vi "Graph.vi"() -> ()   [LabVIEW 2016, in "PanelDataNode.lvclass"]
uses:
  PanelDataNode.lvclass
  PanelObject/PanelObject.lvclass
  PanelDataNode.lvclass/PanelDataNode.ctl
  Split Mode.ctl
  <vilib>/Analysis/baseanly.llb/Mean (DBL).vi
  <vilib>/measure/NI_MABase.lvlib
  <vilib>/Analysis/NI_AALBase.lvlib
panel:
  out "波形图表":waveform(dbl)(graph)={"t0"=timestamp(9406.0 s since 1904-01-01), "dt"=0.001, "Y"=array[1000 elements]}
  in  "Node*":refnum<data-value>
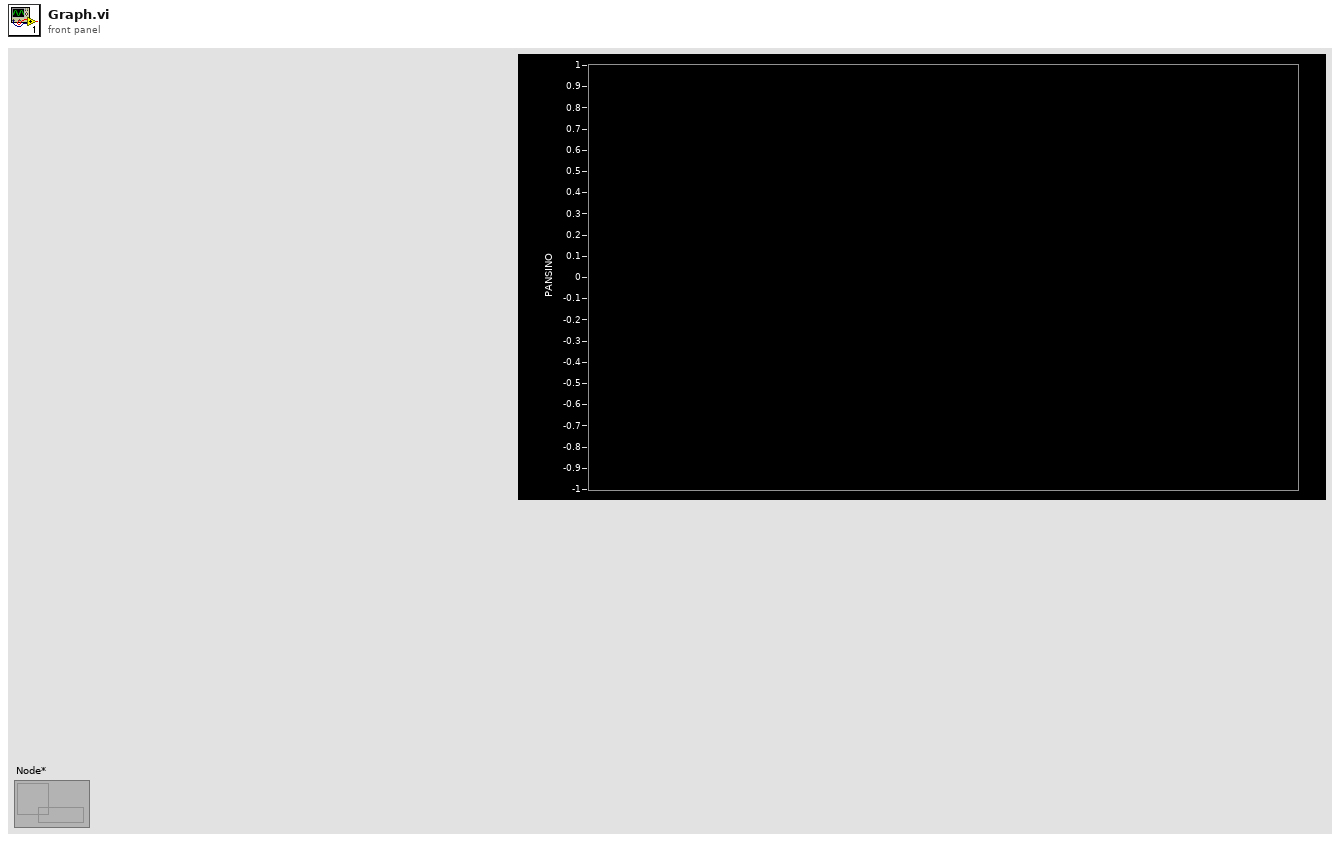
[diagram p1: front panel]
types:
  T1 = enum16{"Sine Wave", "Triangle Wave", "Square Wave", "Sawtooth Wave"}
  T2 = typedef "PanelDataNode.lvclass/Split Mode.ctl" = enum16{"Horizontal(up)", "Vertical(left)", "Horizontal(down)", "Vertical(right)"}
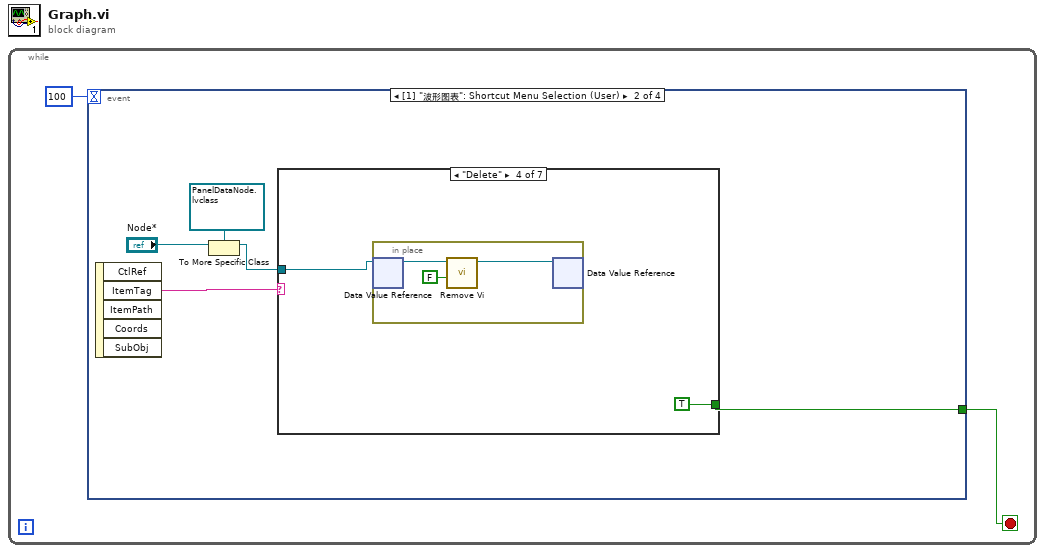
[diagram p0: block diagram]
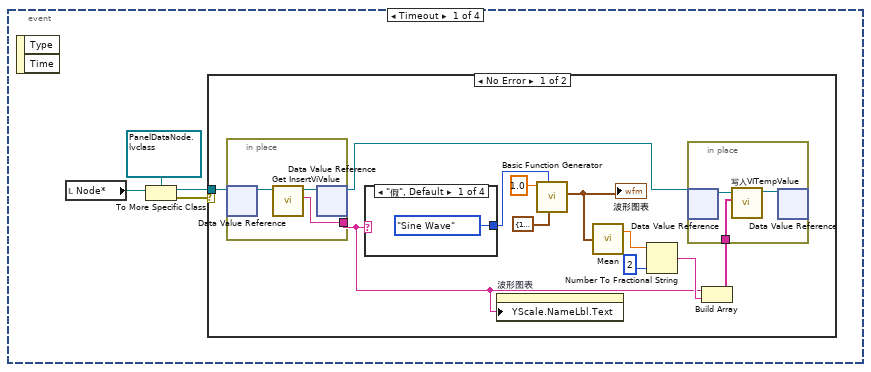
[diagram p2: hidden frame]
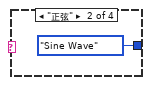
[diagram p3: hidden frame]
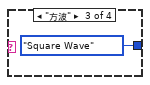
[diagram p4: hidden frame]
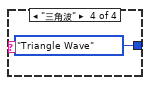
[diagram p5: hidden frame]
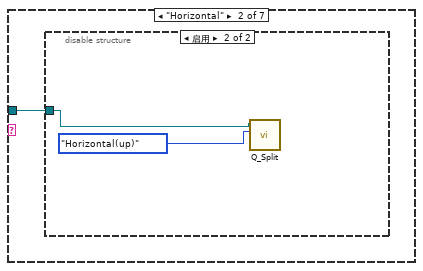
[diagram p8: hidden frame]
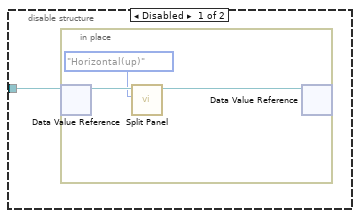
[diagram p9: hidden frame]
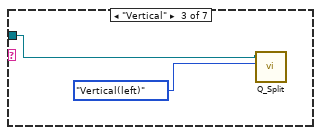
[diagram p10: hidden frame]
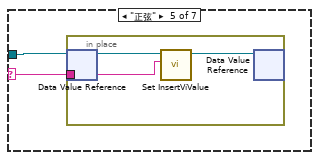
[diagram p11: hidden frame]
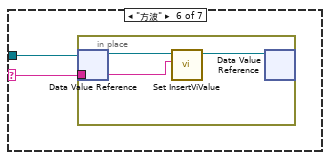
[diagram p12: hidden frame]
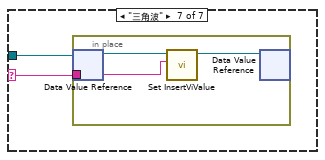
[diagram p13: hidden frame]
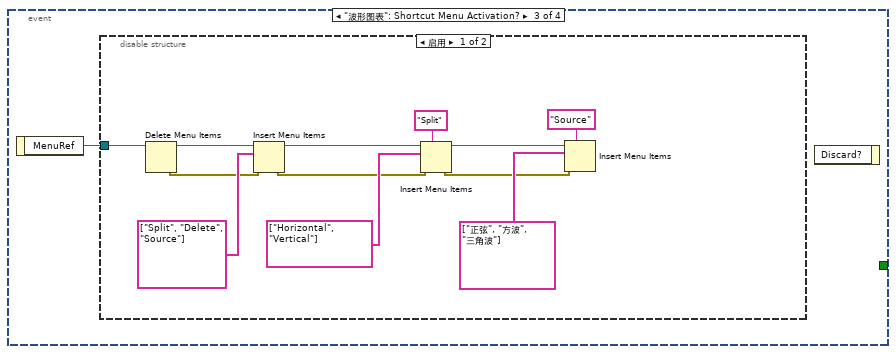
[diagram p14: hidden frame]
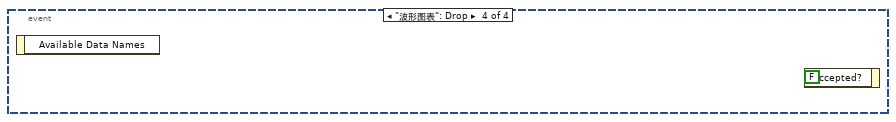
[diagram p16: hidden frame]
diagram:
  n1 = while {
    stop <- w1 stop-if-true
    n2 = event shown="[1] \"波形图表\": Shortcut Menu Selection (User)" {
      selector: _ -> [_ _ _ _]
      dyn-events: _ -> [_ _ _ _]
      timeout: 100 -> [_ _ _ _]
      tunnel: [_ w28 _ _] -> w1
      event Timeout {
        n3 = event-data() -> ()  [unwired: 1 in, 2 out]
        n4 = local read "Node*"() -> (w5:refnum<data-value>)
        n5 = To More Specific Class(target class=refnum<data-value> refnum ("Node*"), reference=w5) -> (specific class reference=w3:refnum<data-value>, error out=w4:errorcluster)  [unwired: 1 in]
        n6 = case shown="No Error" w4 {
          tunnel: w3 -> [w15 _]
          frame No Error {
            n7 = in-place {
              in-place-border: [w25] -> w7
              n8 = in-place-dvr #1(w15) -> (w27:refnum<class "PanelDataNode.lvclass">)  [unwired: 1 out]
              n9 = call-dynamic "Get InsertViValue.vi"("PanelDataNode 输入"=w27) -> ("ViValue"=w25:string, "PanelDataNode 输出"=w26:refnum<class "PanelDataNode.lvclass">)  [unwired: 8 in, 1 out]
              n10 = in-place-dvr #1(w26) -> (w12:refnum<data-value>)  [unwired: 1 out]
            }
            n11 = case shown="\"假\", Default" w7 {
              tunnel: [T1."Sine Wave" ("signal type") T1."Sine Wave" ("signal type") T1."Square Wave" ("signal type") T1."Triangle Wave" ("signal type")] -> w14
              frame "假", Default {
              }
              frame "正弦" {
              }
              frame "方波" {
              }
              frame "三角波" {
              }
            }
            n12 = property on="波形图表" class="WFChart (strict)"("YScale.NameLbl.Text"=w7) -> ()  [unwired: 2 in, 2 out]
            n13 = call <vilib>:"Basic Function Generator.vi"("sampling info"=cluster{"Fs":dbl, "#s":dbl} {"Fs"=100.0, "#s"=101.0}, "signal type"=w14, "frequency"=1.0) -> ("signal out"=w13:waveform(dbl))  [unwired: 6 in, 2 out]
            "波形图表" <- w13
            n14 = call-poly <vilib>:"Mean.vi"("X"=w13) -> ("mean"=w11:dbl)  [unwired: 1 out]
            n15 = Number To Fractional String(number=w11, precision (6)=i16 2 ("精度(6)")) -> (F-format string=w9:string)  [unwired: 2 in]
            n16 = Build Array(w7, w9) -> (w8:string[])
            n17 = in-place {
              in-place-border: w8 -> [w18]
              n18 = in-place-dvr #2(w12) -> (w20:refnum<class "PanelDataNode.lvclass">)  [unwired: 1 out]
              n19 = call "写入VITempValue.vi"("VITempValue"=w18, "PanelDataNode输入"=w20) -> ("PanelDataNode输出"=w19:refnum<class "PanelDataNode.lvclass">)  [unwired: 8 in, 1 out]
              n20 = in-place-dvr #2(w19) -> ()  [unwired: 2 out]
            }
          }
          frame Error {
          }
        }
      }
      event "波形图表": Shortcut Menu Selection (User) {
        n21 = event-data() -> ("ItemTag"=w32:string)  [unwired: 1 in, 4 out]
        n22 = To More Specific Class(target class=refnum<data-value> refnum ("Node*"), reference="Node*") -> (specific class reference=w29:refnum<data-value>)  [unwired: 1 in, 1 out]
        n23 = case shown="\"Delete\"" w32 {
          selector: w32 -> [_ _ _ _ w47 w52 w57]
          tunnel: w29 -> [_ w33 w41 w42 w48 w53 w58]
          tunnel: [_ _ _ TRUE _ _ _] -> w28
          frame "假", Default {
          }
          frame "Horizontal" {
            n24 = disable-structure shown="启用" {
              disable-tunnel: w33 -> [w34 w39]
              frame Disabled {
                n25 = in-place {
                  n26 = in-place-dvr #3(w34) -> (w37:refnum<class "PanelDataNode.lvclass">)  [unwired: 1 out]
                  n27 = call-dynamic "Split Panel.vi"("Split Mode"=Split_Mode."Horizontal(up)", "PanelDataNode 输入"=w37) -> ("PanelDataNode 输出"=w36:refnum<class "PanelDataNode.lvclass">)  [unwired: 7 in, 2 out]
                  n28 = in-place-dvr #3(w36) -> ()  [unwired: 2 out]
                }
              }
              frame Enabled {
                n29 = call "Q_Split.vi"("Split Mode"=Split_Mode."Horizontal(up)", "ChildNode*"=w39) -> ()  [unwired: 9 in, 1 out]
              }
            }
          }
          frame "Vertical" {
            n30 = call "Q_Split.vi"("Split Mode"=Split_Mode."Vertical(left)", "ChildNode*"=w41) -> ()  [unwired: 9 in, 1 out]
          }
          frame "Delete" {
            n31 = in-place {
              n32 = in-place-dvr #4(w42) -> (w46:refnum<class "PanelDataNode.lvclass">)  [unwired: 1 out]
              n33 = call-dynamic "Remove Vi.vi"("Abort VI"=FALSE, "PanelDataNode 输入"=w46) -> ("PanelDataNode 输出"=w45:refnum<class "PanelDataNode.lvclass">)  [unwired: 6 in, 3 out]
              n34 = in-place-dvr #4(w45) -> ()  [unwired: 2 out]
            }
          }
          frame "正弦" {
            n35 = in-place {
              in-place-border: w47 -> [w50]
              n36 = in-place-dvr #5(w48) -> (w51:refnum<class "PanelDataNode.lvclass">)  [unwired: 1 out]
              n37 = call-dynamic "Set InsertViValue.vi"("ViValue"=w50, "PanelDataNode 输入"=w51) -> ("PanelDataNode 输出"=w49:refnum<class "PanelDataNode.lvclass">)  [unwired: 8 in, 1 out]
              n38 = in-place-dvr #5(w49) -> ()  [unwired: 2 out]
            }
          }
          frame "方波" {
            n39 = in-place {
              in-place-border: w52 -> [w55]
              n40 = in-place-dvr #6(w53) -> (w56:refnum<class "PanelDataNode.lvclass">)  [unwired: 1 out]
              n41 = call-dynamic "Set InsertViValue.vi"("ViValue"=w55, "PanelDataNode 输入"=w56) -> ("PanelDataNode 输出"=w54:refnum<class "PanelDataNode.lvclass">)  [unwired: 8 in, 1 out]
              n42 = in-place-dvr #6(w54) -> ()  [unwired: 2 out]
            }
          }
          frame "三角波" {
            n43 = in-place {
              in-place-border: w57 -> [w60]
              n44 = in-place-dvr #7(w58) -> (w61:refnum<class "PanelDataNode.lvclass">)  [unwired: 1 out]
              n45 = call-dynamic "Set InsertViValue.vi"("ViValue"=w60, "PanelDataNode 输入"=w61) -> ("PanelDataNode 输出"=w59:refnum<class "PanelDataNode.lvclass">)  [unwired: 8 in, 1 out]
              n46 = in-place-dvr #7(w59) -> ()  [unwired: 2 out]
            }
          }
        }
      }
      event "波形图表": Shortcut Menu Activation? {
        n47 = event-data() -> ("MenuRef"=w62:refnum<k9>)  [unwired: 1 in]
        n48 = disable-structure shown="启用" {
          disable-tunnel: w62 -> [w74 _]
          frame Enabled {
            n49 = Delete Menu Items(9:w74) -> (0:w65:errorcluster, 3:w73:refnum<k9>)  [unwired: 3 in]
            n50 = Insert Menu Items(6:w65, 8:string[] ["Split", "Delete", "Source"] ("项名称"), 9:w73) -> (0:w64:errorcluster, 3:w71:refnum<k9>)  [unwired: 3 in, 1 out]
            n51 = Insert Menu Items(5:"Split" ("菜单标识符"), 6:w64, 8:string[] ["Horizontal", "Vertical"], 9:w71) -> (0:w63:errorcluster, 3:w68:refnum<k9>)  [unwired: 2 in, 1 out]
            n52 = Insert Menu Items(5:"Source" ("菜单标识符"), 6:w63, 8:string[] ["正弦", "方波", "三角波"] ("项名称"), 9:w68) -> ()  [unwired: 2 in, 3 out]
          }
          frame Disabled {
          }
        }
        n53 = event-data() -> ()  [unwired: 2 in, 1 out]
      }
      event "波形图表": Drop {
        n54 = event-data() -> ()  [unwired: 1 in, 1 out]
        n55 = event-data("Accepted?"=FALSE ("接受？")) -> ()  [unwired: 1 in, 1 out]
      }
    }
  }
